vi "Image.vi"(2 "XRef":refnum<vi>, 3 "State In":T1={"Input Type"=variant(dbl 0.0), "Width"=0, "Typedef Name"="", "Value Type"=variant, "Selection"=0, "Options"=[], "Selections"=[], "Display Selections"=[], "Element Names"=[], "Typedef Name Width"=0, "Display Selection Width"=[], "Code Generated"=FALSE}) -> (0 "Image":picture)   [LabVIEW 2015, in "Read-Write-Signals.xnode"]
doc: "This ability VI is used to describe your XNode's appearance. The origin of Image corresponds to the top-left corner of your XNode. The bounds of your XNode are used to crop this image. If you want LabVIEW to update your image, you need to inform it through the UpdateImage or UpdateImageAndBounds replies. Any areas where you do not draw are transparent, so regions intended to appear white should be explicitly drawn.\n \n Remember to localize any strings that are part of your image.\n\nDefault behavior: None.\n\nThis ability does not provide UI and OS messages are not handled."
uses:
  Read-Write-Signals.xnode
  State.ctl
  Read-Write-Signals Item.ctl
  Read-Write-Signals Sub Item.ctl
  Read-Write-Signals Sub Item Type.ctl
  Read-Write-Signals Selection.ctl
  Read-Write-Signals Display Selection.ctl
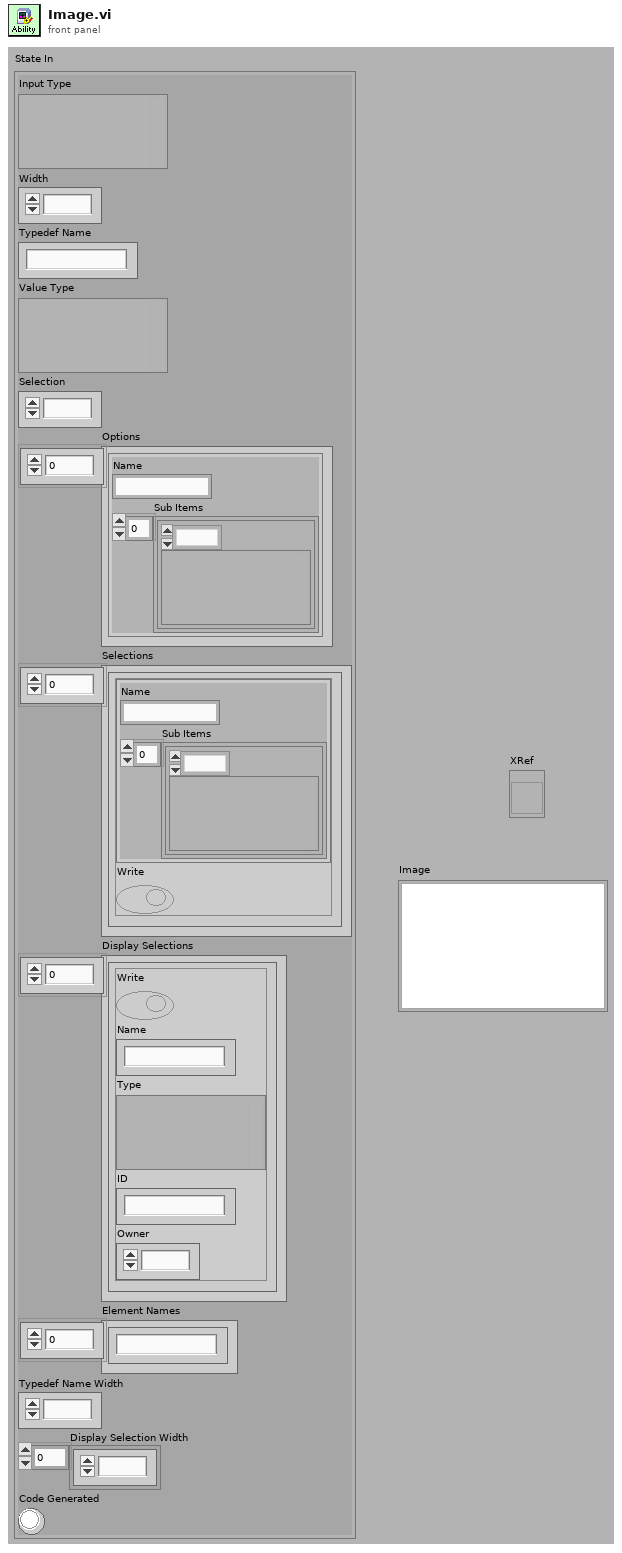
[diagram p1: front panel]
types:
  T1 = typedef "Read-Write-Signals.xnode/State.ctl" = cluster{"Input Type":variant, "Width":i32, "Typedef Name":string, "Value Type":variant, "Selection":i32, "Options":T2[], "Selections":T5[], "Display Selections":T6[], "Element Names":string[], "Typedef Name Width":i32, "Display Selection Width":i32[], "Code Generated":bool}
  T2 = typedef "Read-Write-Signals Item.ctl" = cluster{"Name":string, "Sub Items":T3[]}
  T3 = typedef "Read-Write-Signals Sub Item.ctl" = cluster{"Type":T4, "Value":variant}
  T4 = typedef "Read-Write-Signals Sub Item Type.ctl" = enum8{"Cluster Element", "Array Element", "Subarray"}
  T5 = typedef "Read-Write-Signals Selection.ctl" = cluster{"Item":T2, "Write":bool}
  T6 = typedef "Read-Write-Signals Display Selection.ctl" = cluster{"Write":bool, "Name":string, "Type":variant, "ID":string, "Owner":i32}
  T7 = typedef "imagedata.ctl" = cluster{"image type":i32, "image depth":i32, "image":u8[], "mask":u8[], "colors":u32[], "Rectangle":cluster{"left":i16, "top":i16, "right":i16, "bottom":i16}}
  T8 = cluster{"left":i16, "top":i16, "right":i16, "bottom":i16}
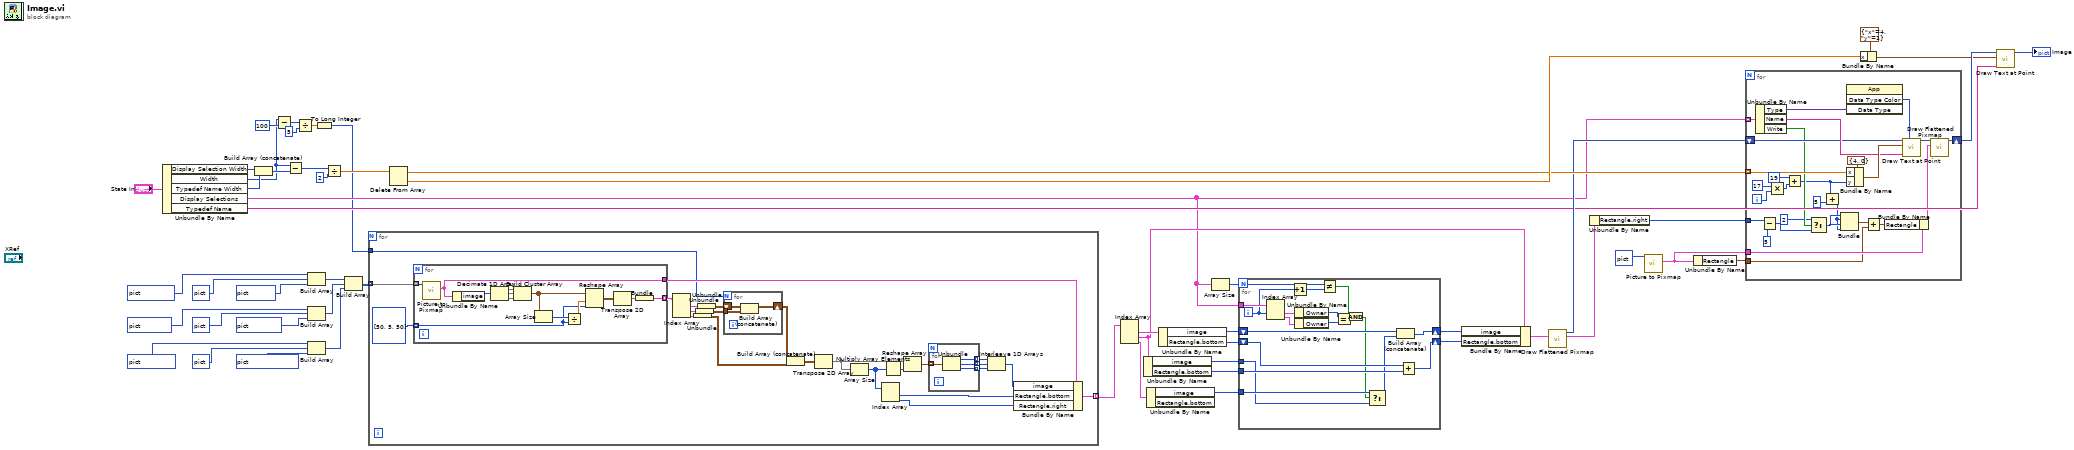
[diagram p0: block diagram]
diagram:
  n1 = Unbundle By Name("State In") -> ("Display Selection Width"=w8:i32[], "Width"=w7:i32, "Typedef Name Width"=w18:i32, "Display Selections"=w2:T6[], "Typedef Name"=w12:string)
  n2 = Build Array (concatenate)(w8, w18) -> (w24:i32[])
  n3 = Subtract(x=w7, y=100) -> (x-y=w29:i32)
  n4 = Subtract(x=w7, y=w24) -> (x-y=w27:i32[])
  n5 = Divide(x=w29, y=i16 5) -> (x/y=w6:dbl)
  n6 = Build Array(picture bytes[2880] ("new picture"), picture bytes[315] ("new picture"), picture bytes[2880] ("new picture")) -> (w43:picture[])
  n7 = Build Array(picture bytes[2580] ("new picture"), picture bytes[285] ("new picture"), picture bytes[2580] ("new picture")) -> (w42:picture[])
  n8 = Build Array(picture bytes[2580] ("new picture"), picture bytes[285] ("new picture"), picture bytes[2580] ("new picture")) -> (w41:picture[])
  n9 = To Long Integer(number=w6) -> (32bit integer=w1:i32)
  n10 = Divide(x=w27, y=i16 2) -> (x/y=w25:dbl[])
  n11 = Build Array(w43, w42, w41) -> (w40:picture[][])
  n12 = for {
    tunnel: w40 -> [w76] mode=indexing
    tunnel: [w57] -> w39 mode=indexing
    tunnel: w1 -> [w53]
    n13 = for {
      tunnel: w76 -> [w96] mode=indexing
      tunnel: i32[] [50, 5, 50] -> [w88] mode=indexing
      tunnel: [w84] -> w74 mode=indexing
      tunnel: [w86] -> w59
      n14 = call <vilib>:"Picture to Pixmap.vi"("picture"=w96) -> ("image data"=w86:T7)  [unwired: 9 in, 1 out]
      n15 = Unbundle By Name(w86) -> ("image"=w92:u8[])
      n16 = Decimate 1D Array(w92) -> (w91:u8[], w89:u8[], w90:u8[])
      n17 = Build Cluster Array(w91, w89, w90) -> (w93:cluster{u8, u8, u8}[])
      n18 = Array Size(array=w93) -> (size(s)=w94:i32)
      n19 = Divide(x=w94, y=w88) -> (x/y=w95:dbl)
      n20 = Reshape Array(w93, w95, w88) -> (w87:cluster{u8, u8, u8}[][])
      n21 = Transpose 2D Array(2D array=w87) -> (transposed array=w85:cluster{u8, u8, u8}[][])
      n22 = Bundle(w85) -> (w84:cluster{cluster{u8, u8, u8}[][]})  [unwired: 1 in]
    }
    n23 = Index Array(array=w74) -> (element #1=w72:cluster{cluster{u8, u8, u8}[][]}, element #2=w73:cluster{cluster{u8, u8, u8}[][]}, element #3=w70:cluster{cluster{u8, u8, u8}[][]})  [unwired: 3 in]
    n24 = Unbundle(w70) -> (w54:cluster{u8, u8, u8}[][])
    n25 = Unbundle(w73) -> (w55:cluster{u8, u8, u8}[][])
    n26 = Unbundle(w72) -> (w56:cluster{u8, u8, u8}[][])
    n27 = for {
      N: w53 -> [_]
      shift-right: [w81] -> w71
      shift-left: w56 -> [w82]
      tunnel: w55 -> [w83]
      n28 = Build Array (concatenate)(w82, w83) -> (w81:cluster{u8, u8, u8}[][])
    }
    n29 = Build Array (concatenate)(w71, w54) -> (w69:cluster{u8, u8, u8}[][])
    n30 = Transpose 2D Array(2D array=w69) -> (transposed array=w60:cluster{u8, u8, u8}[][])
    n31 = Array Size(array=w60) -> (size(s)=w68:i32[])
    n32 = Index Array(array=w68) -> (element #1=w61:i32, element #2=w58:i32)  [unwired: 2 in]
    n33 = Multiply Array Elements(1:w68) -> (0:w67:i32)
    n34 = Reshape Array(w60, w67) -> (w66:cluster{u8, u8, u8}[])
    n35 = for {
      tunnel: w66 -> [w80] mode=indexing
      tunnel: [w79] -> w65 mode=indexing
      tunnel: [w78] -> w64 mode=indexing
      tunnel: [w77] -> w63 mode=indexing
      n36 = Unbundle(w80) -> (w79:u8, w78:u8, w77:u8)
    }
    n37 = Interleave 1D Arrays(w65, w64, w63) -> (w62:u8[])
    n38 = Bundle By Name(cluster=w59, "image"=w62, "Rectangle.bottom"=w61, "Rectangle.right"=w58) -> (w57:T7)
  }
  n39 = Delete From Array(array=w25) -> (deleted portion=w17:dbl, array with subset deleted=w16:dbl[])  [unwired: 2 in]
  n40 = Index Array(array=w39) -> (element #1=w38:T7, element #2=w33:T7, element #3=w5:T7)  [unwired: 3 in]
  n41 = Unbundle By Name(w33) -> ("image"=w36:u8[], "Rectangle.bottom"=w35:i16)
  n42 = Unbundle By Name(w5) -> ("image"=w4:u8[])  [unwired: 1 out]
  n43 = Unbundle By Name(w38) -> ("image"=w37:u8[], "Rectangle.bottom"=w34:i16)
  n44 = Array Size(array=w2) -> (size(s)=w3:i32)
  n45 = for {
    N: w3 -> [w99]
    tunnel: w36 -> [w103]
    tunnel: w35 -> [w114]
    shift-right: [w111] -> w31
    shift-left: w37 -> [w115]
    shift-right: [w112] -> w32
    shift-left: w34 -> [w113]
    tunnel: w2 -> [w110]
    tunnel: w4 -> [w104]
    i -> [w97]
    n46 = Index Array(array=w110, index #1=w97) -> (element #1=w109:T6, element #2=w108:T6)  [unwired: 1 in]
    n47 = Increment(x=w97) -> (x+1=w98:i32)
    n48 = Unbundle By Name(w109) -> ("Owner"=w107:i32)
    n49 = Unbundle By Name(w108) -> ("Owner"=w106:i32)
    n50 = Not Equal?(x=w99, y=w98) -> (x != y?=w100:bool)
    n51 = Equal?(x=w107, y=w106) -> (x = y?=w105:bool)
    n52 = And(x=w100, y=w105) -> (x .and. y?=w101:bool)
    n53 = Select(t=w104, s=w101, f=w103) -> (s? t:f=w102:u8[])
    n54 = Build Array (concatenate)(w115, w102) -> (w111:u8[])
    n55 = Add(x=w113, y=w114) -> (x+y=w112:i16)
  }
  n56 = Bundle By Name(cluster=w33, "image"=w31, "Rectangle.bottom"=w32) -> (w13:T7)
  n57 = call <vilib>:"Draw Flattened Pixmap.vi"("image data"=w13) -> ("new picture"=w15:picture)  [unwired: 1 in, 7 out]
  n58 = Unbundle By Name(w13) -> ("Rectangle.right"=w20:i16)
  n59 = call <vilib>:"Picture to Pixmap.vi"("picture"=picture bytes[84] ("new picture")) -> ("image data"=w9:T7)  [unwired: 9 in, 1 out]
  n60 = Unbundle By Name(w9) -> ("Rectangle"=w19:T8)
  n61 = for {
    tunnel: w2 -> [w137] mode=indexing
    shift-right: [w132] -> w23
    shift-left: w15 -> [w135]
    tunnel: w16 -> [w134] mode=indexing
    tunnel: w20 -> [w130]
    tunnel: w19 -> [w124]
    tunnel: w9 -> [w131]
    i -> [w141]
    n62 = Unbundle By Name(w137) -> ("Type"=w116:variant, "Name"=w136:string, "Write"=w128:bool)
    n63 = Subtract(x=w130, y=i16 5) -> (x-y=w127:i16)
    n64 = Multiply(x=17, y=w141) -> (x*y=w139:i32)
    n65 = Add(x=19, y=w139) -> (x+y=w120:i32)
    n66 = Select(t=i16 2 ("y"), s=w128, f=w127) -> (s? t:f=w125:i16)
    n67 = Add(x=w120, y=5) -> (x+y=w119:i32)
    n68 = Bundle("y"=w125, w119, "y"=w125, w119) -> (w123:cluster{"y":i16, i32, "y":i16, i32})  [unwired: 1 in]
    n69 = invoke class="App" method="Data Type Color"("Data Type"=w116) -> ("Data Type Color"=w117:u32)  [unwired: 3 in, 3 out]
    n70 = Bundle By Name(cluster=cluster{"x":i16, "y":i16} {"x"=4, "y"=0} ("origin"), "x"=w134, "y"=w120) -> (w142:cluster{"x":i16, "y":i16})
    n71 = Add(x=w123, y=w124) -> (x+y=w122:cluster{i16, i32, i16, i32})
    n72 = Bundle By Name(cluster=w131, "Rectangle"=w122) -> (w121:T7)
    n73 = call <vilib>:"Draw Text at Point.vi"("text color(black)"=w117, "text"=w136, "origin"=w142, "picture"=w135) -> ("new picture"=w133:picture)  [unwired: 6 in, 1 out]
    n74 = call <vilib>:"Draw Flattened Pixmap.vi"("image data"=w121, "picture"=w133) -> ("new picture"=w132:picture)  [unwired: 7 out]
  }
  n75 = Bundle By Name(cluster=cluster{"x":i16, "y":i16} {"x"=4, "y"=1} ("origin"), "x"=w17) -> (w21:cluster{"x":i16, "y":i16})
  n76 = call <vilib>:"Draw Text at Point.vi"("text"=w12, "origin"=w21, "picture"=w23) -> ("new picture"=→"Image":picture)  [unwired: 7 in, 1 out]
